vi "Calculate_bottle_distance_matrix_multicolor.vi"(8 "Monomolecular":string[](array[string]), 9 "Odour bottles":T1(array[cluster]), 10 "Mixture":string[](array[string]), 11 "XYGraph in":refnum<vi>) -> (3 "appended array":cluster{"MDS1":dbl[], "MDS2":dbl[]}[](array[cluster]))   [LabVIEW 2016]
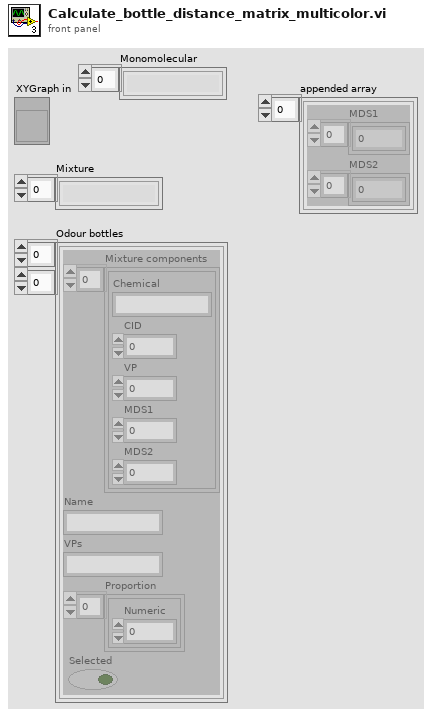
[diagram p1: front panel]
types:
  T1 = cluster{"Mixture components":cluster{"Chemical":string, "CID":i32, "VP":dbl, "MDS1":dbl, "MDS2":dbl}[], "Name":string, "VPs":string, "Proportion":cluster{"Numeric":dbl}[], "Selected":bool}[][]
  T2 = cluster{"Mixture components":cluster{"Chemical":string, "CID":i32, "VP":dbl, "MDS1":dbl, "MDS2":dbl}[], "Name":string, "VPs":string, "Proportion":cluster{"Numeric":dbl}[], "Selected":bool}[]
  T3 = cluster{"Chemical":string, "CID":i32, "VP":dbl, "MDS1":dbl, "MDS2":dbl}[]
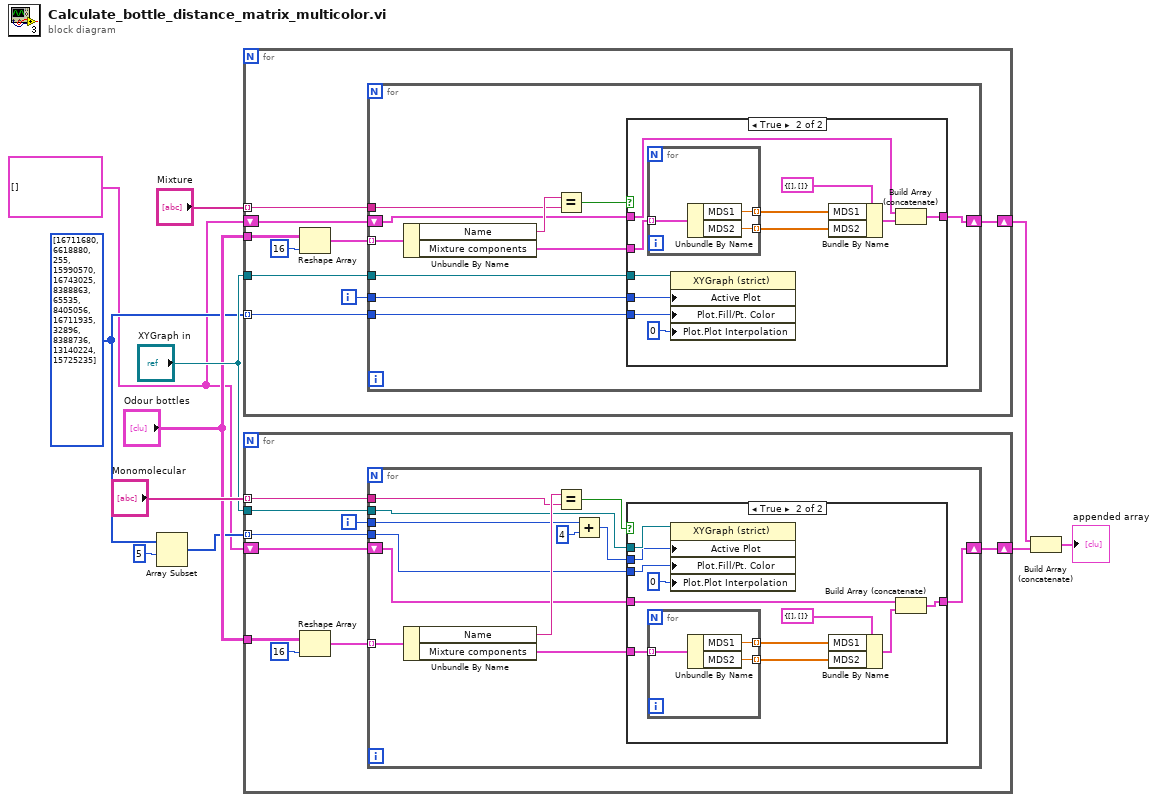
[diagram p0: block diagram]
diagram:
  w1 = cluster{"MDS1":dbl[], "MDS2":dbl[]}[] [] ("appended array")
  w6 = u32[] [16711680, 6618880, 255, 15990570, 16743025, 8388863, 65535, 8405056, 16711935, 32896, 8388736, 13140224, 15725235]
  n1 = Array Subset(array=w6, index=5) -> (w4:u32[])  [unwired: 1 in]
  n2 = for {
    tunnel: "Mixture" -> [w17] mode=indexing
    tunnel: w6 -> [w14] mode=indexing
    tunnel: "Odour bottles" -> [w20]
    shift-right: [w15] -> w11
    shift-left: w1 -> [w16]
    tunnel: "XYGraph in" -> [w12]
    i -> [w13]
    n3 = Reshape Array(w20, 16 ("dimension size")) -> (w18:T2)
    n4 = for {
      tunnel: w18 -> [w30] mode=indexing
      tunnel: w17 -> [w28]
      shift-right: [w25] -> w15
      shift-left: w16 -> [w26]
      tunnel: w14 -> [w23]
      tunnel: w13 -> [w22]
      tunnel: w12 -> [w21]
      n5 = Unbundle By Name(w30) -> ("Name"=w29:string, "Mixture components"=w24:T3)
      n6 = Equal?(x=w29, y=w28) -> (x = y?=w27:bool)
      n7 = case shown="True" w27 {
        tunnel: w26 -> [w31 w40]
        tunnel: [w31 w39] -> w25
        tunnel: w24 -> [_ w42]
        tunnel: w23 -> [_ w35]
        tunnel: w22 -> [_ w34]
        tunnel: w21 -> [_ w32]
        frame False {
        }
        frame True {
          n8 = for {
            tunnel: w42 -> [w45] mode=indexing
            tunnel: [w44] -> w37 mode=indexing
            tunnel: [w43] -> w36 mode=indexing
            n9 = Unbundle By Name(w45) -> ("MDS1"=w44:dbl, "MDS2"=w43:dbl)
          }
          n10 = property on="Property Node" class="XYGraph (strict)"(reference=w32, "Active Plot"=w34, "Plot.Fill/Pt. Color"=w35, "Plot.Plot Interpolation"=u8 0) -> ()  [unwired: 1 in, 2 out]
          n11 = Bundle By Name(cluster=cluster{"MDS1":dbl[], "MDS2":dbl[]} {"MDS1"=[], "MDS2"=[]} ("input cluster"), "MDS1"=w37, "MDS2"=w36) -> (w38:cluster{"MDS1":dbl[], "MDS2":dbl[]})
          n12 = Build Array (concatenate)(w40, w38) -> (w39:cluster{"MDS1":dbl[], "MDS2":dbl[]}[])
        }
      }
    }
  }
  n13 = for {
    tunnel: "Monomolecular" -> [w51] mode=indexing
    tunnel: w4 -> [w48] mode=indexing
    tunnel: "Odour bottles" -> [w54]
    shift-right: [w49] -> w2
    shift-left: w1 -> [w50]
    tunnel: "XYGraph in" -> [w46]
    i -> [w47]
    n14 = Reshape Array(w54, 16 ("dimension size")) -> (w52:T2)
    n15 = for {
      tunnel: w52 -> [w66] mode=indexing
      tunnel: w51 -> [w64]
      shift-right: [w61] -> w49
      shift-left: w50 -> [w62]
      tunnel: w48 -> [w59]
      tunnel: w47 -> [w58]
      tunnel: w46 -> [w57]
      n16 = Unbundle By Name(w66) -> ("Name"=w65:string, "Mixture components"=w60:T3)
      n17 = Equal?(x=w65, y=w64) -> (x = y?=w63:bool)
      n18 = Add(x=w58, y=4) -> (x+y=w56:i32)
      n19 = case shown="True" w63 {
        tunnel: w62 -> [w67 w76]
        tunnel: [w67 w75] -> w61
        tunnel: w60 -> [_ w78]
        tunnel: w59 -> [_ w71]
        tunnel: w56 -> [_ w68]
        tunnel: w57 -> [_ w69]
        frame False {
        }
        frame True {
          n20 = for {
            tunnel: w78 -> [w81] mode=indexing
            tunnel: [w80] -> w73 mode=indexing
            tunnel: [w79] -> w72 mode=indexing
            n21 = Unbundle By Name(w81) -> ("MDS1"=w80:dbl, "MDS2"=w79:dbl)
          }
          n22 = property on="Property Node" class="XYGraph (strict)"(reference=w69, "Active Plot"=w68, "Plot.Fill/Pt. Color"=w71, "Plot.Plot Interpolation"=u8 0) -> ()  [unwired: 1 in, 2 out]
          n23 = Bundle By Name(cluster=cluster{"MDS1":dbl[], "MDS2":dbl[]} {"MDS1"=[], "MDS2"=[]} ("input cluster"), "MDS1"=w73, "MDS2"=w72) -> (w74:cluster{"MDS1":dbl[], "MDS2":dbl[]})
          n24 = Build Array (concatenate)(w76, w74) -> (w75:cluster{"MDS1":dbl[], "MDS2":dbl[]}[])
        }
      }
    }
  }
  n25 = Build Array (concatenate)(w11, w2) -> (→"appended array":cluster{"MDS1":dbl[], "MDS2":dbl[]}[])
